vi "DAQmx.44xx.Fs to FilterDelay.vi"(8 "error in (no error)":errorcluster, 11 "Refnum in":refnum<k21>) -> (0 "error out":errorcluster, 1 "DAC Delay (samples)":dbl, 2 "ADC Delay (samples)":dbl, 3 "Refnum out":refnum<k21>, 4 "Total Filter Delay (samples)":dbl)   [LabVIEW 2019, in "DAQmx.lvclass"]
uses:
  DAQmx.lvclass
  <resource>/objmgr/daqmx.rc
panel:
  out "SampClk.Rate":dbl format="%_27g"
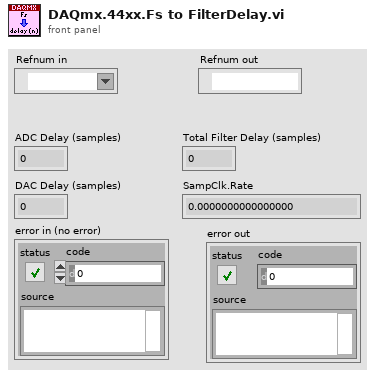
[diagram p1: front panel]
types:
  T1 = typedef "DAQmx.lvclass/DAQ.Config.Device Type--enum.ctl" = enum16{"None", "USB-4431", "PXI-446x"}
  T2 = enum16{"1.0 <= fs <= 1.6", "1.6 < fs <= 3.2", "3.2 < fs <= 6.4", "6.4 < fs <= 12.8", "12.8 < fs <= 25.6", "25.6 < fs <= 51.2", "51.2 < fs <= 102.4", "102.4 < fs <= 204.8"}
  T3 = enum16{"0.8 <= fs <= 1.6", "1.6 < fs <= 3.2", "3.2 < fs <= 6.4", "6.4 < fs <= 12.8", "12.8 < fs <= 25.6", "25.6 < fs <= 51.2", "51.2 < fs <= 102.4"}
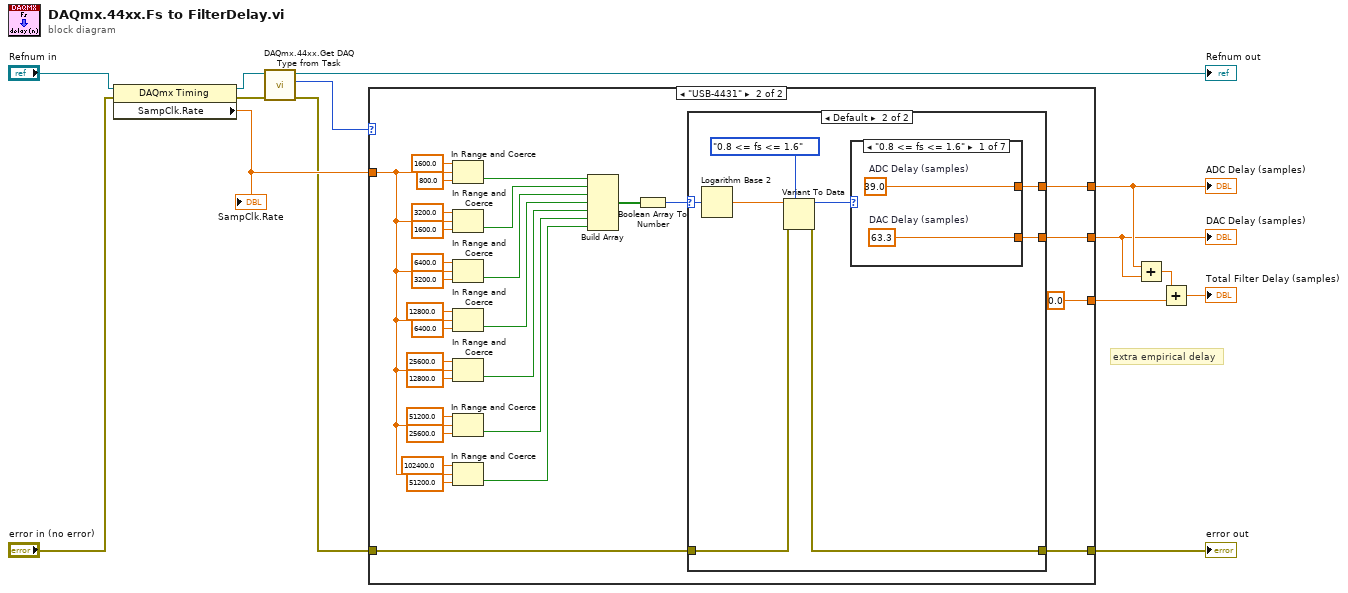
[diagram p0: block diagram]
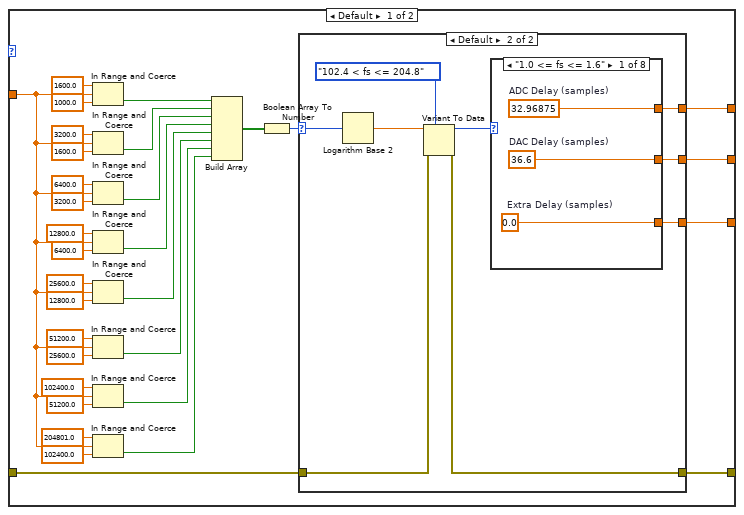
[diagram p2: hidden frame]
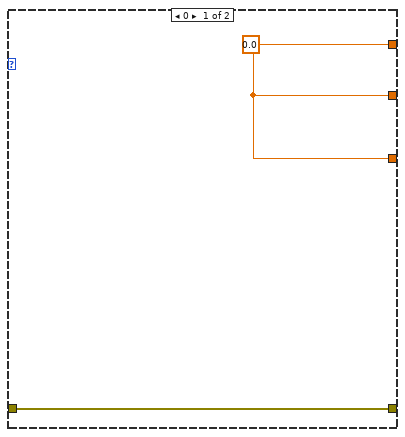
[diagram p3: hidden frame]
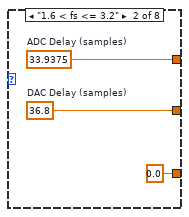
[diagram p4: hidden frame]
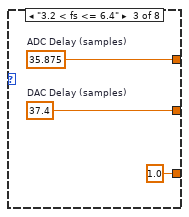
[diagram p5: hidden frame]
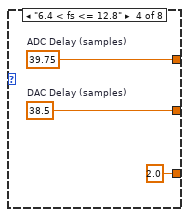
[diagram p6: hidden frame]
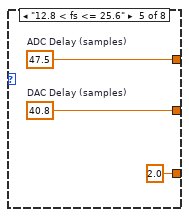
[diagram p7: hidden frame]
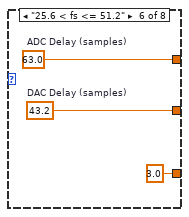
[diagram p8: hidden frame]
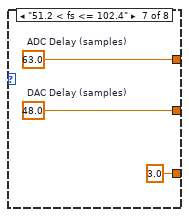
[diagram p9: hidden frame]
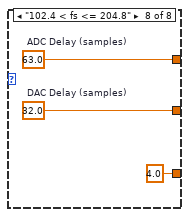
[diagram p10: hidden frame]
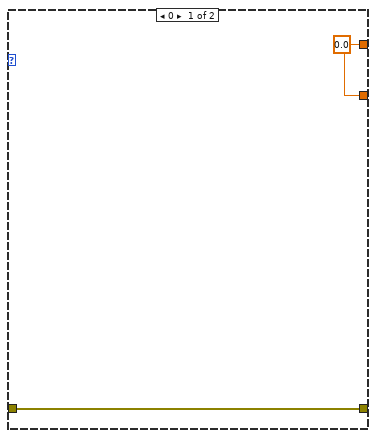
[diagram p11: hidden frame]
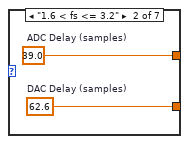
[diagram p12: hidden frame]
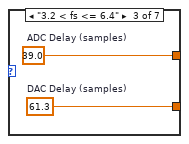
[diagram p13: hidden frame]
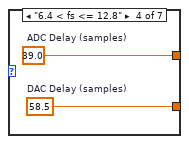
[diagram p14: hidden frame]
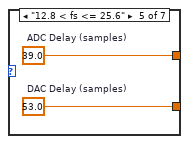
[diagram p15: hidden frame]
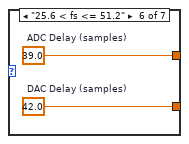
[diagram p16: hidden frame]
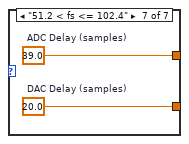
[diagram p17: hidden frame]
diagram:
  # "extra empirical delay"
  n1 = property class="DAQmx Timing"(reference="Refnum in", error in="error in (no error)") -> (reference out=w13:refnum<k21>, error out=w11:errorcluster, "SampClk.Rate"=w5:dbl)
  "SampClk.Rate" <- w5
  n2 = call "DAQmx.44xx.Get DAQ Type from Task.vi"("error in (no error)"=w11, "Task in"=w13) -> ("error out"=w4:errorcluster, "DAQ Type"=w6:T1, "Task out"=→"Refnum out":refnum<k21>)  [unwired: 5 in, 2 out]
  n3 = case shown="\"USB-4431\"" w6 {
    tunnel: w5 -> [w30 w96]
    tunnel: [w20 w87] -> w8
    tunnel: [w19 w86] -> w9
    tunnel: w4 -> [w18 w85]
    tunnel: [w17 w84] -> w7
    tunnel: [w15 0.0 ("Extra Delay (samples)")] -> w1
    frame Default {
      n4 = In Range and Coerce(upper limit=1600.0, x=w30, lower limit=1000.0) -> (In Range?=w29:bool)  [unwired: 1 out]
      n5 = In Range and Coerce(upper limit=3200.0, x=w30, lower limit=1600.0) -> (In Range?=w28:bool)  [unwired: 1 out]
      n6 = In Range and Coerce(upper limit=6400.0, x=w30, lower limit=3200.0) -> (In Range?=w27:bool)  [unwired: 1 out]
      n7 = In Range and Coerce(upper limit=12800.0, x=w30, lower limit=6400.0) -> (In Range?=w26:bool)  [unwired: 1 out]
      n8 = In Range and Coerce(upper limit=25600.0, x=w30, lower limit=12800.0) -> (In Range?=w25:bool)  [unwired: 1 out]
      n9 = In Range and Coerce(upper limit=51200.0, x=w30, lower limit=25600.0) -> (In Range?=w24:bool)  [unwired: 1 out]
      n10 = In Range and Coerce(upper limit=102400.0, x=w30, lower limit=51200.0) -> (In Range?=w23:bool)  [unwired: 1 out]
      n11 = In Range and Coerce(upper limit=204801.0, x=w30, lower limit=102400.0) -> (In Range?=w22:bool)  [unwired: 1 out]
      n12 = Build Array(w29, w28, w27, w26, w25, w24, w23, w22) -> (w21:bool[])
      n13 = Boolean Array To Number(Boolean array=w21) -> (number=w16:u32)
      n14 = case shown="Default" w16 {
        selector: w16 -> [_ w50]
        tunnel: [w47 w56] -> w20
        tunnel: [w47 w55] -> w19
        tunnel: w18 -> [w48 w53]
        tunnel: [w48 w52] -> w17
        tunnel: [w47 w49] -> w15
        frame 0 {
          w47 = 0.0 ("ADC Delay (samples)")
        }
        frame Default {
          n15 = Logarithm Base 2(1:w50) -> (0:w51:dbl)
          n16 = Variant To Data(error in=w53, type=T2."102.4 < fs <= 204.8", Variant=w51) -> (data=w54:T2, error out=w52:errorcluster)
          n17 = case shown="\"1.0 <= fs <= 1.6\"" w54 {
            tunnel: [w60 w63 w66 w69 w72 w75 w78 w81] -> w55
            tunnel: [w59 w62 w65 w68 w71 w74 w77 w80] -> w56
            tunnel: [w58 0.0 ("Extra Delay (samples)") 1.0 ("Extra Delay (samples)") 2.0 ("Extra Delay (samples)") 2.0 ("Extra Delay (samples)") 3.0 ("Extra Delay (samples)") 3.0 ("Extra Delay (samples)") 4.0 ("Extra Delay (samples)")] -> w49
            frame "1.0 <= fs <= 1.6" {
              w58 = 0.0  # Extra Delay (samples)
              w59 = 36.6  # DAC Delay (samples)
              w60 = 32.96875  # ADC Delay (samples)
            }
            frame "1.6 < fs <= 3.2" {
              w62 = 36.8  # DAC Delay (samples)
              w63 = 33.9375  # ADC Delay (samples)
            }
            frame "3.2 < fs <= 6.4" {
              w65 = 37.4  # DAC Delay (samples)
              w66 = 35.875  # ADC Delay (samples)
            }
            frame "6.4 < fs <= 12.8" {
              w68 = 38.5  # DAC Delay (samples)
              w69 = 39.75  # ADC Delay (samples)
            }
            frame "12.8 < fs <= 25.6" {
              w71 = 40.8  # DAC Delay (samples)
              w72 = 47.5  # ADC Delay (samples)
            }
            frame "25.6 < fs <= 51.2" {
              w75 = 63.0  # ADC Delay (samples)
              w74 = 43.2  # DAC Delay (samples)
            }
            frame "51.2 < fs <= 102.4" {
              w78 = 63.0  # ADC Delay (samples)
              w77 = 48.0  # DAC Delay (samples)
            }
            frame "102.4 < fs <= 204.8" {
              w81 = 63.0  # ADC Delay (samples)
              w80 = 32.0  # DAC Delay (samples)
            }
          }
        }
      }
    }
    frame "USB-4431" {
      n18 = In Range and Coerce(upper limit=1600.0, x=w96, lower limit=800.0) -> (In Range?=w95:bool)  [unwired: 1 out]
      n19 = In Range and Coerce(upper limit=3200.0, x=w96, lower limit=1600.0) -> (In Range?=w94:bool)  [unwired: 1 out]
      n20 = In Range and Coerce(upper limit=6400.0, x=w96, lower limit=3200.0) -> (In Range?=w93:bool)  [unwired: 1 out]
      n21 = In Range and Coerce(upper limit=12800.0, x=w96, lower limit=6400.0) -> (In Range?=w92:bool)  [unwired: 1 out]
      n22 = In Range and Coerce(upper limit=25600.0, x=w96, lower limit=12800.0) -> (In Range?=w91:bool)  [unwired: 1 out]
      n23 = In Range and Coerce(upper limit=51200.0, x=w96, lower limit=25600.0) -> (In Range?=w90:bool)  [unwired: 1 out]
      n24 = In Range and Coerce(upper limit=102400.0, x=w96, lower limit=51200.0) -> (In Range?=w89:bool)  [unwired: 1 out]
      n25 = Build Array(w95, w94, w93, w92, w91, w90, w89) -> (w88:bool[])
      n26 = Boolean Array To Number(Boolean array=w88) -> (number=w83:u32)
      n27 = case shown="Default" w83 {
        selector: w83 -> [_ w114]
        tunnel: [w112 w120] -> w87
        tunnel: [w112 w119] -> w86
        tunnel: w85 -> [w111 w116]
        tunnel: [w111 w115] -> w84
        frame 0 {
          w112 = 0.0 ("ADC Delay (samples)")
        }
        frame Default {
          n28 = Logarithm Base 2(1:w114) -> (0:w113:dbl)
          n29 = Variant To Data(error in=w116, type=T3."0.8 <= fs <= 1.6", Variant=w113) -> (data=w117:T3, error out=w115:errorcluster)
          n30 = case shown="\"0.8 <= fs <= 1.6\"" w117 {
            tunnel: [w122 w124 w126 w128 w130 w132 w134] -> w119
            tunnel: [w121 w123 w125 w127 w129 w131 w133] -> w120
            frame "0.8 <= fs <= 1.6" {
              w121 = 63.3  # DAC Delay (samples)
              w122 = 39.0  # ADC Delay (samples)
            }
            frame "1.6 < fs <= 3.2" {
              w123 = 62.6  # DAC Delay (samples)
              w124 = 39.0  # ADC Delay (samples)
            }
            frame "3.2 < fs <= 6.4" {
              w125 = 61.3  # DAC Delay (samples)
              w126 = 39.0  # ADC Delay (samples)
            }
            frame "6.4 < fs <= 12.8" {
              w127 = 58.5  # DAC Delay (samples)
              w128 = 39.0  # ADC Delay (samples)
            }
            frame "12.8 < fs <= 25.6" {
              w129 = 53.0  # DAC Delay (samples)
              w130 = 39.0  # ADC Delay (samples)
            }
            frame "25.6 < fs <= 51.2" {
              w132 = 39.0  # ADC Delay (samples)
              w131 = 42.0  # DAC Delay (samples)
            }
            frame "51.2 < fs <= 102.4" {
              w134 = 39.0  # ADC Delay (samples)
              w133 = 20.0  # DAC Delay (samples)
            }
          }
        }
      }
    }
  }
  "error out" <- w7
  "ADC Delay (samples)" <- w9
  "DAC Delay (samples)" <- w8
  n31 = Add(x=w9, y=w8) -> (x+y=w3:dbl)
  n32 = Add(x=w3, y=w1) -> (x+y=→"Total Filter Delay (samples)":dbl)
